vi "AlliGator Parse Version History reStructuredText File Content.vi"(8 "Error In":errorcluster, 9 "Current Version Number":string, 11 "Version History Page rst body":string) -> (0 "Error Out":errorcluster, 1 "Latest Version":string, 2 "Release Date":string, 3 "New in this Version":string, 5 "Version up to date":bool)   [LabVIEW 2021, in "AlliGator GUI.lvlib"]
doc: "Gets the version history page from the ReadTheDocs manual page and extracts the \"New in this version\" text for the last version."
uses:
  AlliGator GUI.lvlib
  Strings/Strings.lvlib
  Utilities/Utilities.lvlib
panel:
  # "see the AlliGator License on the block diagram (Ctrl+E or Window:Show Block Diagram)"
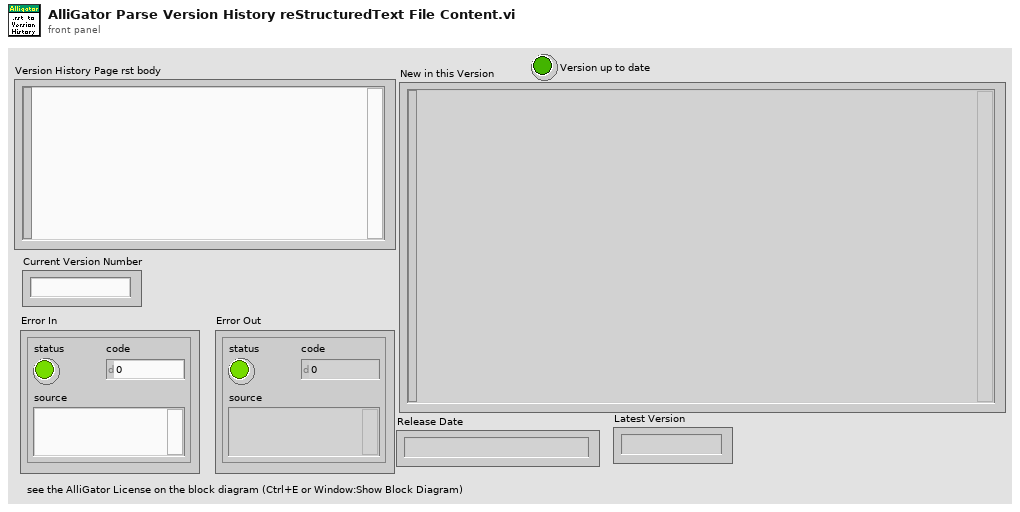
[diagram p1: front panel]
types:
  T1 = typedef "Utilities.lvlib/Version Description.ctl" = cluster{"Major Version Number":i32, "Minor Version Number":i32, "Revision Number":i32, "Version Type":T2, "a/b/rc/ Version Number":i32}
  T2 = typedef "Utilities.lvlib/Version Type.ctl" = enum16{"alpha", "beta", "release candidate", "release"}
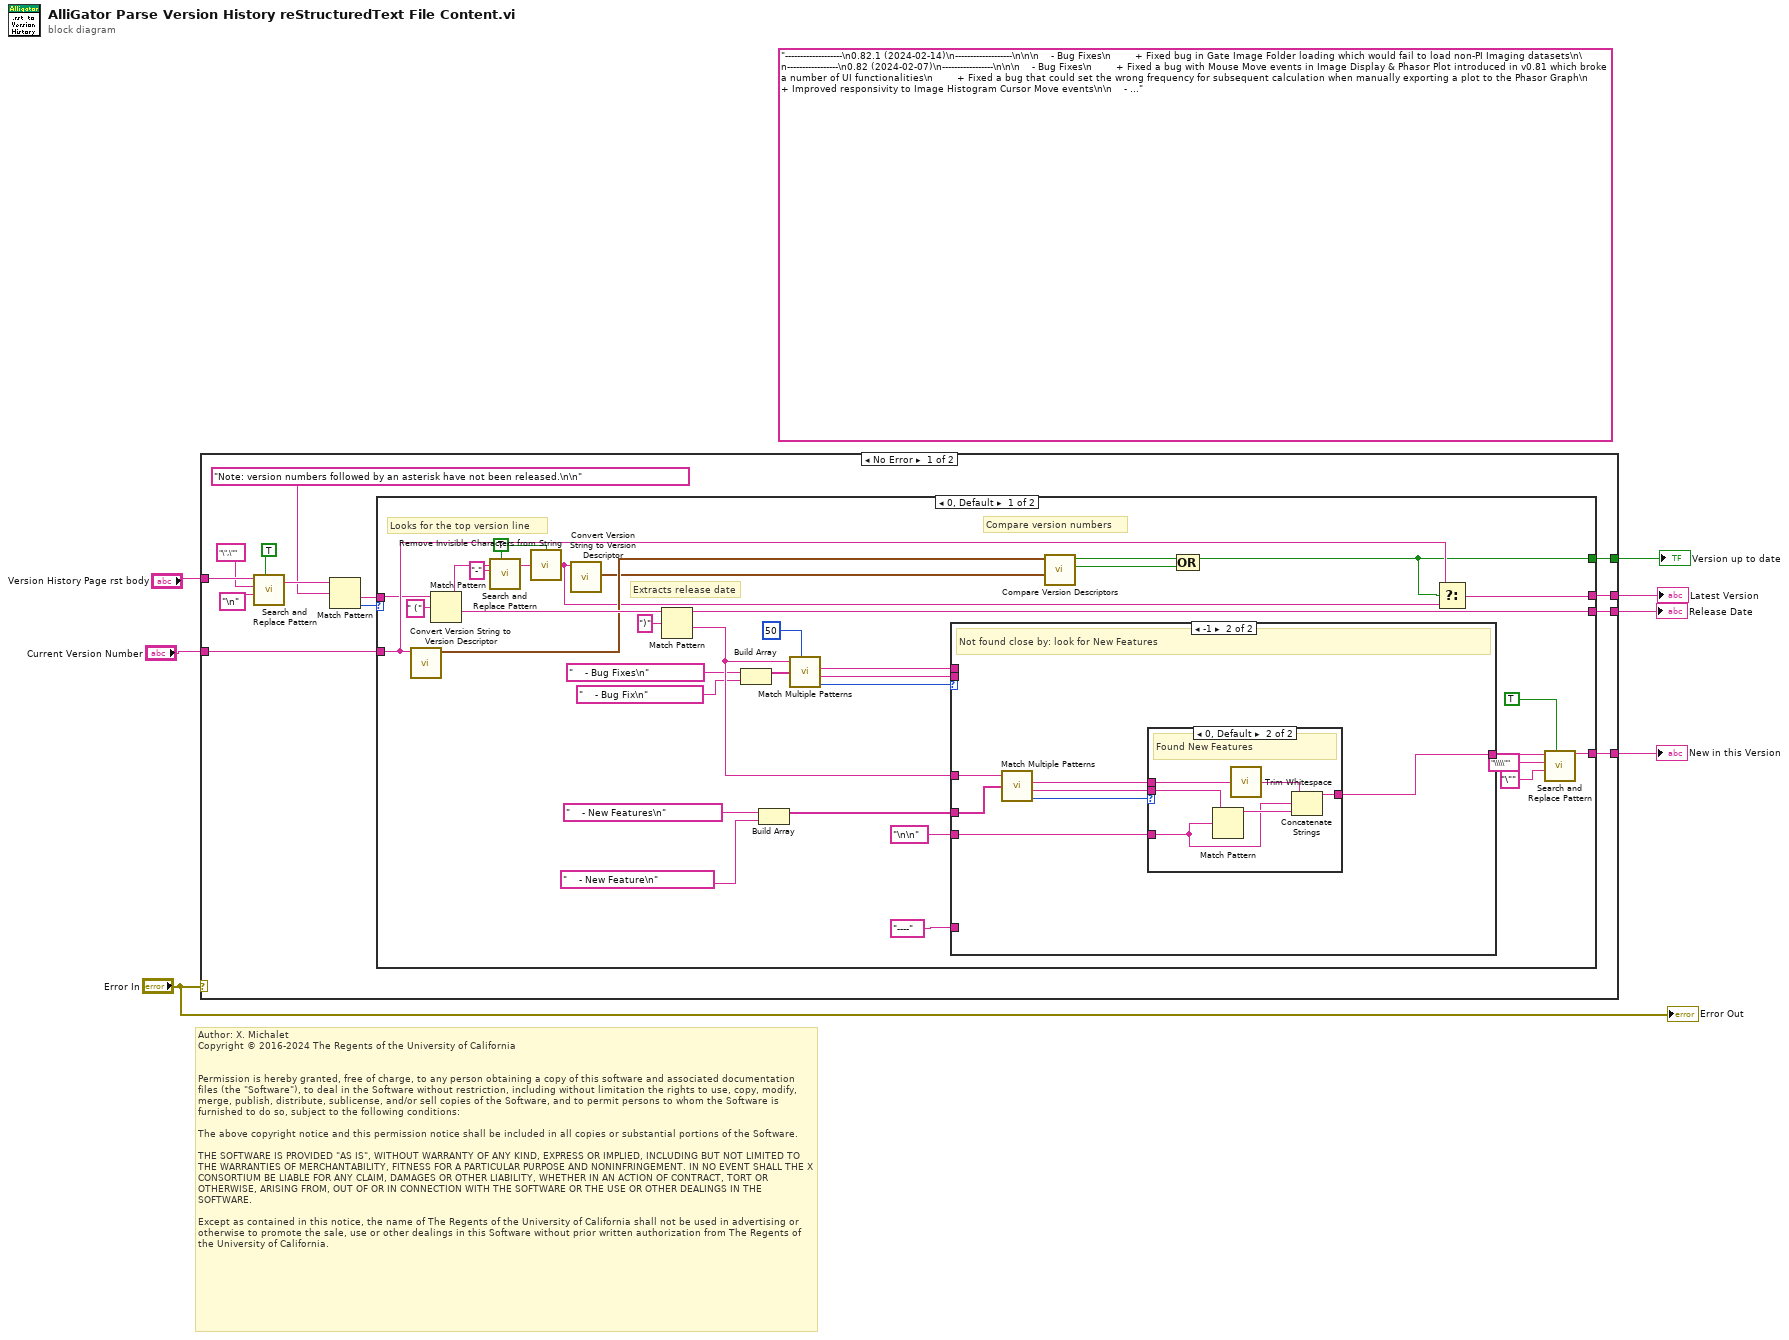
[diagram p0: block diagram]
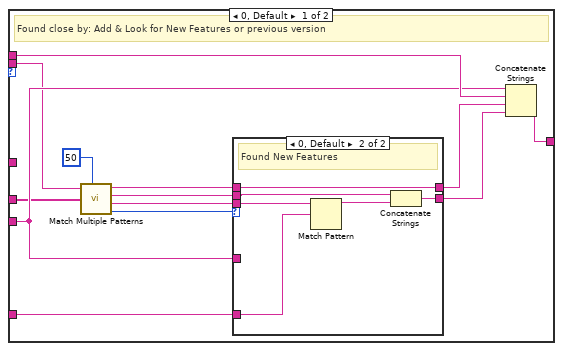
[diagram p2: hidden frame]
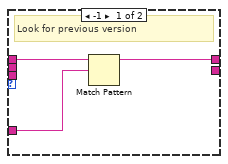
[diagram p3: hidden frame]
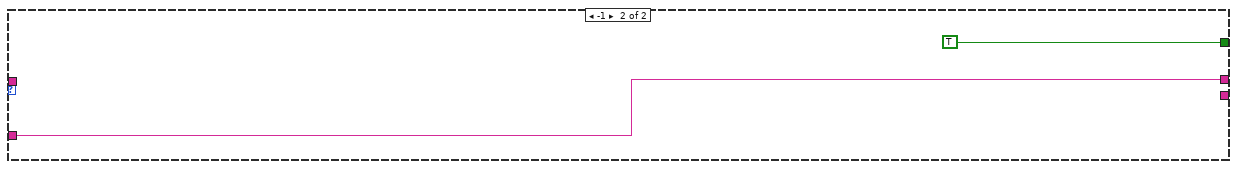
[diagram p5: hidden frame]
diagram:
  (unwired) "-------------------\n0.82.1 (2024-02-14)\n-------------------\n\n\n    - Bug Fixes\n        + Fixed bug in Gate Image Folder loading which would fail to load non-PI Imaging datasets\n\n-----------------\n0.82 (2024-02-07)\n-----------------\n\n\n    - Bug Fixes\n        + Fixed a bug with Mouse Move events in Image Display & Phasor Plot introduced in v0.81 which broke a number of UI functionalities\n        + Fixed a bug that could set the wrong frequency for subsequent calculation when manually exporting a plot to the Phasor Graph\n        + Improved responsivity to Image Histogram Cursor Move events\n\n    - New Features\n        + Added \"Shot Noise Influence on Average Lifetime\" to the Analysis>>Tools menu\n        + Deprecated \"Simple Search\" algorithm when using the Phasor Calibration Map option\n        + Added Dialog allowing to use the frequency of the calibration phasor (or phasor map/phasor series) if it is different from the  current phasor frequency\n\n-----------------\n0.81 (2024-02-03)\n-----------------"
  # "Author: X. Michalet\nCopyright © 2016-2024 The Regents of the University of California\n \n\nPermission is hereby granted, free of charge, to any person obtaining a copy of this software and associated documentation files (the \"Software\"), to deal in the Software without restriction, including without limitation the rights to use, copy, modify, merge, publish, distribute, sublicense, and/or sell copies of the Software, and to permit persons to whom the Software is furnished to do so, subject to the following conditions:\n\nThe above copyright notice and this permission notice shall be included in all copies or substantial portions of the Software.\n\nTHE SOFTWARE IS PROVIDED \"AS IS\", WITHOUT WARRANTY OF ANY KIND, EXPRESS OR IMPLIED, INCLUDING BUT NOT LIMITED TO THE WARRANTIES OF MERCHANTABILITY, FITNESS FOR A PARTICULAR PURPOSE AND NONINFRINGEMENT. IN NO EVENT SHALL THE X CONSORTIUM BE LIABLE FOR ANY CLAIM, DAMAGES OR OTHER LIABILITY, WHETHER IN AN ACTION OF CONTRACT, TORT OR OTHERWISE, ARISING FROM, OUT OF OR IN CONNECTION WITH THE SOFTWARE OR THE USE OR OTHER DEALINGS IN THE SOFTWARE.\n\nExcept as contained in this notice, the name of The Regents of the University of California shall not be used in advertising or otherwise to promote the sale, use or other dealings in this Software without prior written authorization from The Regents of the University of California."
  n1 = case shown="No Error" "Error In" {
    tunnel: [w20 _] -> w7
    tunnel: [w19 _] -> w6
    tunnel: [w18 _] -> w5
    tunnel: "Version History Page rst body" -> [w17 _]
    tunnel: "Current Version Number" -> [w14 _]
    tunnel: [w8 _] -> w1
    frame No Error {
      n2 = call <vilib>:"Search and Replace Pattern.vi"("string"=w17, "regular expression (\"\")"="\",\"" ("regular expression (\"\")"), "replace string (\"\")"="\n" ("replace string (\"\")"), "replace all? (F)"=TRUE) -> ("result string"=w13:string)  [unwired: 1 in, 1 out]
      n3 = Match Pattern(string=w13, regular expression="Note: version numbers followed by an asterisk have not been released.\n\n") -> (after substring=w9:string, offset past match=w11:i32)  [unwired: 1 in, 2 out]
      n4 = case shown="0, Default" w11 {
        tunnel: [w48 _] -> w20
        tunnel: [w52 _] -> w19
        tunnel: [w44 w92] -> w18
        tunnel: w14 -> [w42 w92]
        tunnel: w9 -> [w41 _]
        tunnel: [w32 TRUE] -> w8
        frame 0, Default {
          w34 = TRUE ("replace all? (F)")
          # "Compare version numbers"
          # "Extracts release date"
          # "Looks for the top version line"
          n5 = call "Convert Version String to Version Descriptor.vi"("Version Number (String)"=w42) -> ("Version Description"=w40:T1)  [unwired: 9 in, 1 out]
          n6 = Match Pattern(string=w41, regular expression=" (") -> (before substring=w37:string, after substring=w54:string)  [unwired: 1 in, 2 out]
          n7 = call <vilib>:"Search and Replace Pattern.vi"("string"=w37, "regular expression (\"\")"="-" ("regular expression (\"\")"), "replace all? (F)"=w34) -> ("result string"=w36:string)  [unwired: 2 in, 1 out]
          n8 = call "Remove Invisible Characters from String.vi"("Remove Line Feed. etc (F)"=w34, "String"=w36) -> ("result string"=w33:string)  [unwired: 2 in]
          n9 = call "Convert Version String to Version Descriptor.vi"("Version Number (String)"=w33) -> ("Version Description"=w39:T1)  [unwired: 9 in, 1 out]
          n10 = Match Pattern(string=w54, regular expression=")") -> (before substring=w52:string, after substring=w30:string)  [unwired: 1 in, 2 out]
          n11 = Build Array("    - Bug Fixes\n" ("regular expression"), "    - Bug Fix\n" ("regular expression")) -> (w26:string[])
          n12 = Build Array("    - New Features\n" ("regular expression"), "    - New Feature\n" ("regular expression")) -> (w23:string[])
          n13 = call "Match Multiple Patterns.vi"("string"=w30, "upper limit (Inf)"=50, "regular expression"=w26) -> ("match substring"=w29:string, "after substring"=w28:string, "offset past match"=w24:i32)  [unwired: 3 in, 2 out]
          n14 = case shown="-1" w24 {
            tunnel: [w67 w83] -> w49
            tunnel: w30 -> [_ w82]
            tunnel: w28 -> [w62 _]
            tunnel: w23 -> [w61 w81]
            tunnel: "\n\n" ("regular expression") -> [w63 w84]
            tunnel: w29 -> [w64 _]
            tunnel: "----" ("string") -> [w65 _]
            frame 0, Default {
              # "Found close by: Add & Look for New Features or previous version"
              n15 = call "Match Multiple Patterns.vi"("string"=w62, "upper limit (Inf)"=50, "regular expression"=w61) -> ("before substring"=w60:string, "match substring"=w59:string, "after substring"=w58:string, "offset past match"=w57:i32)  [unwired: 3 in, 1 out]
              n16 = case shown="0, Default" w57 {
                tunnel: [_ w77] -> w68
                tunnel: w58 -> [_ w73]
                tunnel: w63 -> [w71 _]
                tunnel: w60 -> [w70 w75]
                tunnel: [w69 w75] -> w66
                tunnel: w59 -> [_ w72]
                tunnel: w65 -> [_ w74]
                frame -1 {
                  # "Look for previous version"
                  n17 = Match Pattern(string=w70, regular expression=w71) -> (before substring=w69:string)  [unwired: 1 in, 3 out]
                }
                frame 0, Default {
                  # "Found New Features"
                  n18 = Match Pattern(string=w73, regular expression=w74) -> (before substring=w76:string)  [unwired: 1 in, 3 out]
                  n19 = Concatenate Strings(w72, w76) -> (w77:string)
                }
              }
              n20 = Concatenate Strings(w63, w64, w66, w68) -> (w67:string)
            }
            frame -1 {
              # "Not found close by: look for New Features"
              n21 = call "Match Multiple Patterns.vi"("string"=w82, "regular expression"=w81) -> ("match substring"=w79:string, "after substring"=w78:string, "offset past match"=w80:i32)  [unwired: 4 in, 2 out]
              n22 = case shown="0, Default" w80 {
                tunnel: [_ w90] -> w83
                tunnel: w78 -> [_ w89]
                tunnel: w84 -> [_ w85]
                tunnel: w79 -> [_ w86]
                frame -1 {
                  # "not found"
                }
                frame 0, Default {
                  # "Found New Features"
                  n23 = Match Pattern(string=w89, regular expression=w85) -> (before substring=w88:string)  [unwired: 1 in, 3 out]
                  n24 = call <vilib>:"Trim Whitespace.vi"("string"=w86) -> ("trimmed string"=w87:string)  [unwired: 1 in]
                  n25 = Concatenate Strings(w87, w85, w88) -> (w90:string)
                }
              }
            }
          }
          n26 = call "Compare Version Descriptors.vi"("Version Description 2"=w39, "Version Description 1"=w40) -> ("Version 1 = Version 2"=w31:bool, "Version 1 > Version 2"=w38:bool)  [unwired: 7 in, 1 out]
          n27 = Compound Arithmetic op=OR(w38, w31) -> (w32:bool)
          n28 = Select(t=w42, s=w32, f=w33) -> (s? t:f=w44:string)
          n29 = call <vilib>:"Search and Replace Pattern.vi"("string"=w49, "regular expression (\"\")"="\\\\\"" ("regular expression (\"\")"), "replace string (\"\")"="\"" ("replace string (\"\")"), "replace all? (F)"=TRUE) -> ("result string"=w48:string)  [unwired: 1 in, 1 out]
        }
        frame -1 {
        }
      }
    }
    frame Error {
    }
  }
  "New in this Version" <- w7
  "Release Date" <- w6
  "Version up to date" <- w1
  "Latest Version" <- w5
  "Error Out" <- "Error In"
